vi "Temp,Hum.vi"() -> ()   [LabVIEW 2017]
uses:
  <vilib>/Instr/_visa.llb/VISA Configure Serial Port (Instr).vi
  <vilib>/express/express shared/transition.llb/Dynamic To Waveform Array.vi
  <vilib>/express/express signal manip/GetorSetDDTAttributes/Set DDT Attributes/SetT0.vi
  <vilib>/express/express shared/transition.llb/Waveform Array To Dynamic.vi
  <vilib>/express/express signal manip/GetorSetDDTAttributes/Set DDT Attributes/Set DDT Properties.xnode
panel:
  out "?":bool
  out "Humidity 3":dbl(slide) scale=0.0..100.0
  out "Temperature 3":dbl(slide) scale=0.0..100.0
  out "?":bool
  out "?":cluster{dbl, dbl}(graph)
  out "Raw Data":string
  out "?":bool
  out "?":bool
  out "?":bool
  out "?":bool
  in  "?":bool
  out "Humidity 2":dbl(slide) scale=0.0..100.0
  out "Humidity 1":dbl(slide) scale=0.0..100.0
  out "Temperature 2":dbl(slide) scale=0.0..100.0
  in  "VISA resource name":refnum<visa-resource-name>
  out "Temperature 1":dbl(slide) scale=0.0..100.0
  out "Waveform Chart":cluster{dbl, dbl, dbl, dbl}(graph)
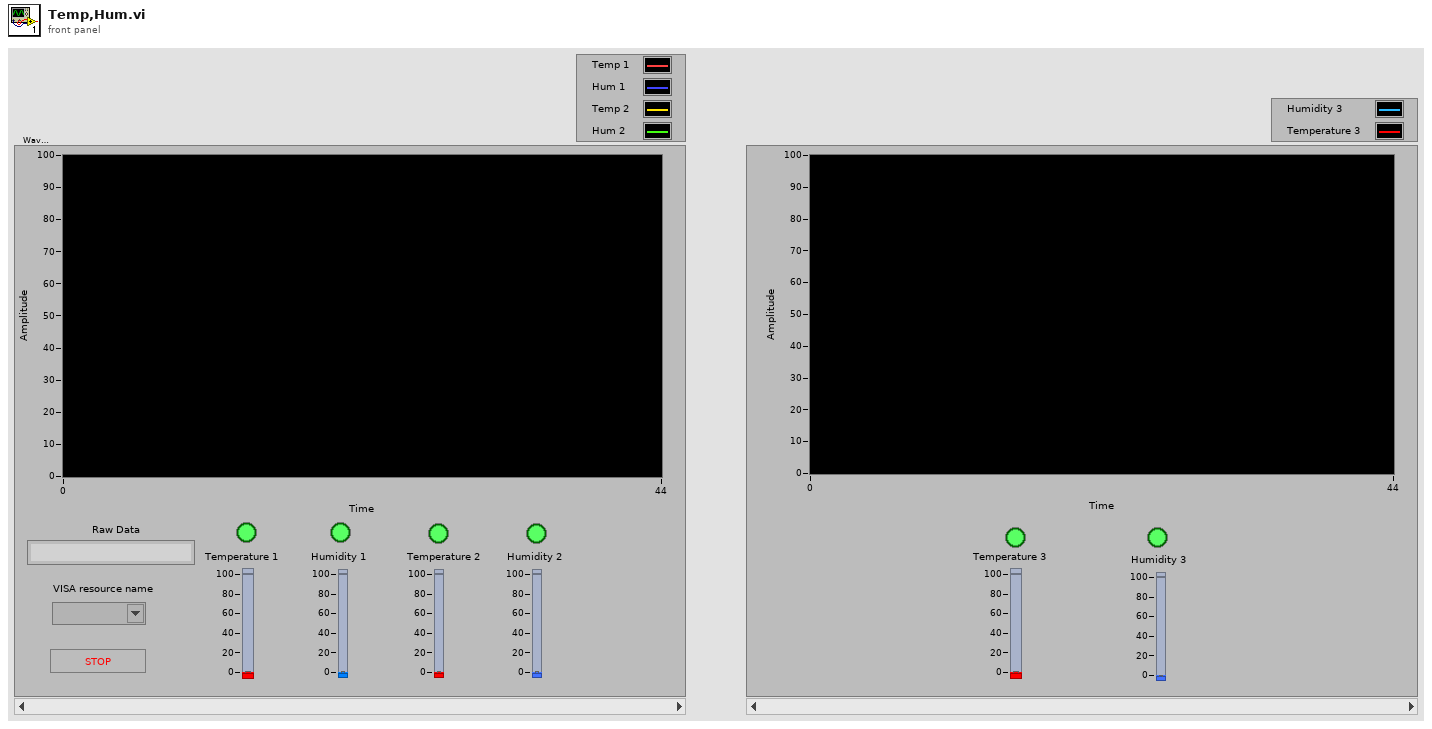
[diagram p1: front panel]
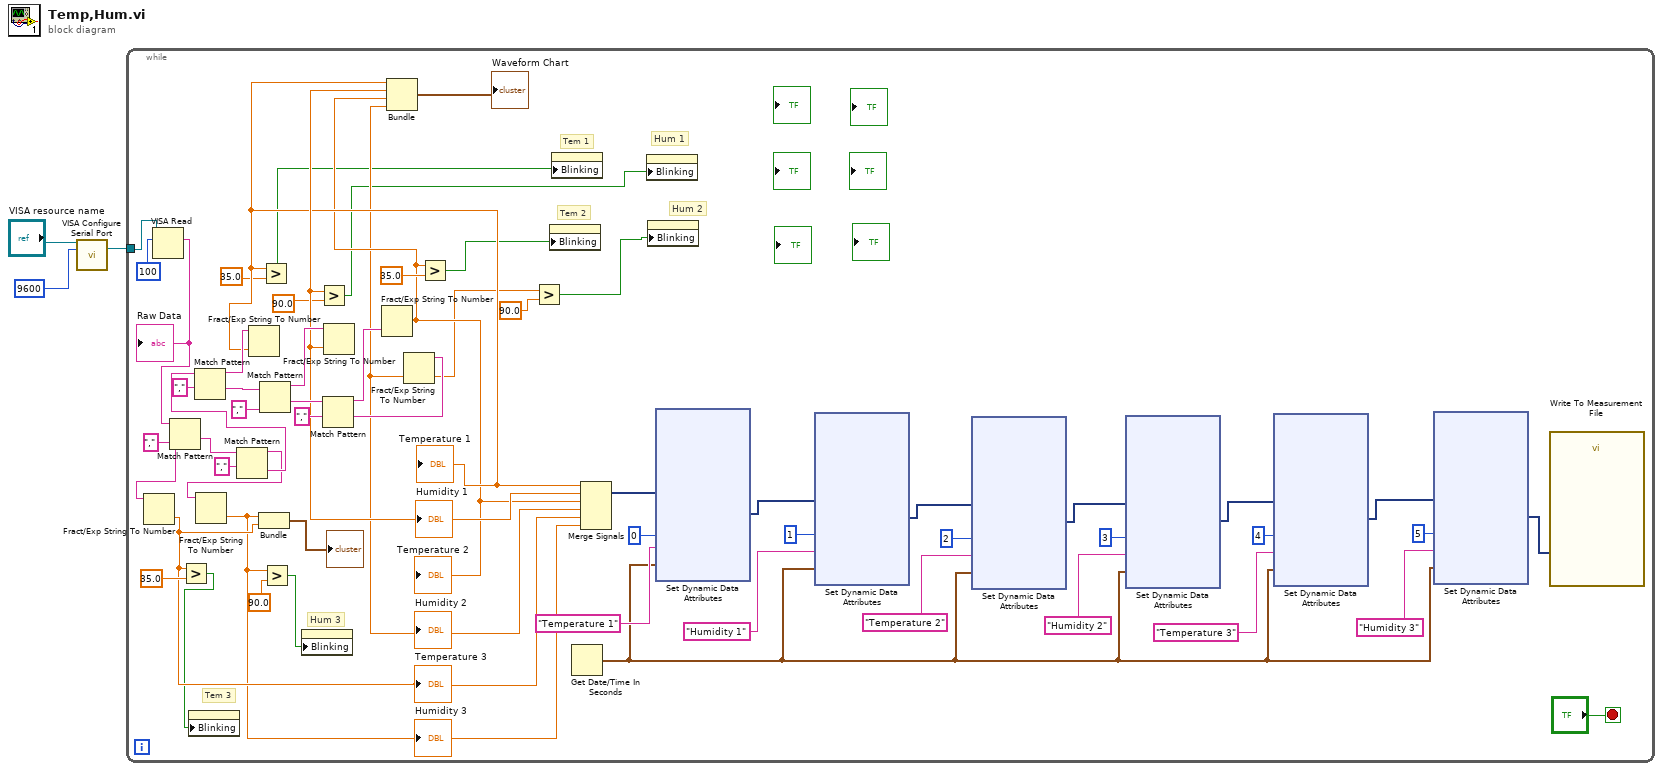
[diagram p0: block diagram]
diagram:
  n1 = call-poly "VISA Configure Serial Port"("VISA resource name"="VISA resource name", "baud rate (9600)"=u32 9600) -> ("VISA resource name out"=w3:refnum<visa-resource-name>)  [unwired: 12 in, 1 out]
  n2 = while {
    tunnel: w3 -> [w62]
    stop <- "?" stop-if-true
    # "Hum 3"
    # "Hum 2"
    # "Tem 2"
    # "Tem 3"
    # "Hum 1"
    # "Tem 1"
    n3 = VISA Read(VISA resource name=w62, byte count=u32 100) -> (read buffer=w29:string)  [unwired: 1 in, 3 out]
    "Raw Data" <- w29
    n4 = Match Pattern(string=w29, regular expression=",") -> (before substring=w25:string, after substring=w27:string)  [unwired: 1 in, 2 out]
    n5 = Fract/Exp String To Number(string=w25) -> (number=w12:dbl)  [unwired: 3 in, 1 out]
    "Temperature 3" <- w12
    n6 = Greater?(x=w12, y=35.0) -> (0:w5:bool)
    n7 = property class="Bool (strict)"("Blinking"=w5) -> ()  [unwired: 2 in, 2 out]
    n8 = Match Pattern(string=w27, regular expression=",") -> (before substring=w24:string, after substring=w26:string)  [unwired: 1 in, 2 out]
    n9 = Match Pattern(string=w26, regular expression=",") -> (before substring=w54:string, after substring=w58:string)  [unwired: 1 in, 2 out]
    n10 = Fract/Exp String To Number(string=w24) -> (number=w11:dbl)  [unwired: 3 in, 1 out]
    "Humidity 3" <- w11
    n11 = Fract/Exp String To Number(string=w54) -> (number=w35:dbl)  [unwired: 3 in, 1 out]
    "Temperature 1" <- w35
    n12 = Bundle(w11, w12) -> (→"?":cluster{dbl, dbl})  [unwired: 1 in]
    n13 = Match Pattern(string=w58, regular expression=",") -> (before substring=w53:string, after substring=w56:string)  [unwired: 1 in, 2 out]
    n14 = Greater?(x=w35, y=35.0) -> (0:w9:bool)
    n15 = Greater?(x=w11, y=90.0) -> (0:w4:bool)
    n16 = property class="Bool (strict)"("Blinking"=w4) -> ()  [unwired: 2 in, 2 out]
    n17 = Match Pattern(string=w56, regular expression=",") -> (before substring=w37:string, after substring=w52:string)  [unwired: 1 in, 2 out]
    n18 = Fract/Exp String To Number(string=w53) -> (number=w36:dbl)  [unwired: 3 in, 1 out]
    "Humidity 1" <- w36
    n19 = Greater?(x=w36, y=90.0) -> (0:w8:bool)
    n20 = Fract/Exp String To Number(string=w37) -> (number=w31:dbl)  [unwired: 3 in, 1 out]
    "Temperature 2" <- w31
    n21 = Fract/Exp String To Number(string=w52) -> (number=w15:dbl)  [unwired: 3 in, 1 out]
    "Humidity 2" <- w15
    n22 = Bundle(w35, w36, w31, w15) -> (→"Waveform Chart":cluster{dbl, dbl, dbl, dbl})  [unwired: 1 in]
    n23 = Greater?(x=w31, y=35.0) -> (0:w7:bool)
    n24 = Greater?(x=w15, y=90.0) -> (0:w6:bool)
    n25 = property class="Bool (strict)"("Blinking"=w7) -> ()  [unwired: 2 in, 2 out]
    n26 = property class="Bool (strict)"("Blinking"=w9) -> ()  [unwired: 2 in, 2 out]
    n27 = Get Date/Time In Seconds() -> (seconds since 1Jan1904=w10:timestamp)
    n28 = Merge Signals(w35, w36, w31, w15, w12, w11) -> (w41:dynamicdata)
    n29 = property class="Bool (strict)"("Blinking"=w8) -> ()  [unwired: 2 in, 2 out]
    n30 = property class="Bool (strict)"("Blinking"=w6) -> ()  [unwired: 2 in, 2 out]
    n31 = xnode "Set Dynamic Data Attributes"("Signals In"=w41, "Signal Index"=0, "Signal Name"="Temperature 1", "Timestamp"=w10) -> ("Signals Out"=w47:dynamicdata)  [unwired: 1 in, 1 out]
    n32 = xnode "Set Dynamic Data Attributes"("Signals In"=w47, "Signal Index"=1, "Signal Name"="Humidity 1", "Timestamp"=w10) -> ("Signals Out"=w38:dynamicdata)  [unwired: 1 in, 1 out]
    n33 = xnode "Set Dynamic Data Attributes"("Signals In"=w38, "Signal Index"=2, "Signal Name"="Temperature 2", "Timestamp"=w10) -> ("Signals Out"=w39:dynamicdata)  [unwired: 1 in, 1 out]
    n34 = xnode "Set Dynamic Data Attributes"("Signals In"=w39, "Signal Index"=3, "Signal Name"="Humidity 2", "Timestamp"=w10) -> ("Signals Out"=w22:dynamicdata)  [unwired: 1 in, 1 out]
    n35 = xnode "Set Dynamic Data Attributes"("Signals In"=w22, "Signal Index"=4, "Signal Name"="Temperature 3", "Timestamp"=w10) -> ("Signals Out"=w20:dynamicdata)  [unwired: 1 in, 1 out]
    n36 = xnode "Set Dynamic Data Attributes"("Signals In"=w20, "Signal Index"=5, "Signal Name"="Humidity 3", "Timestamp"=w10) -> ("Signals Out"=w16:dynamicdata)  [unwired: 1 in, 1 out]
    n37 = call "Write To Measurement File"("Signals"=w16) -> ()  [unwired: 16 in, 3 out]
  }
